vi "Modbus Engine.vi"() -> ()   [LabVIEW 2011]
uses:
  Tushars Events/Software/Modules/EventClient_ObjectReference.ctl
  Strict Type Controls/Settings Operation.ctl
  VIs/MOD bus/nimodbus121/nimodbus121/86/vi.lib/NI Modbus.llb/MB Serial Master Query Write Single Register (poly).vi
  VIs/MOD bus/nimodbus121/nimodbus121/86/vi.lib/NI Modbus.llb/MB Serial Master Query Read Input Registers (poly).vi
panel:
  out "Quit":bool
  out "error out":errorcluster
  in  "error in (no error)":errorcluster
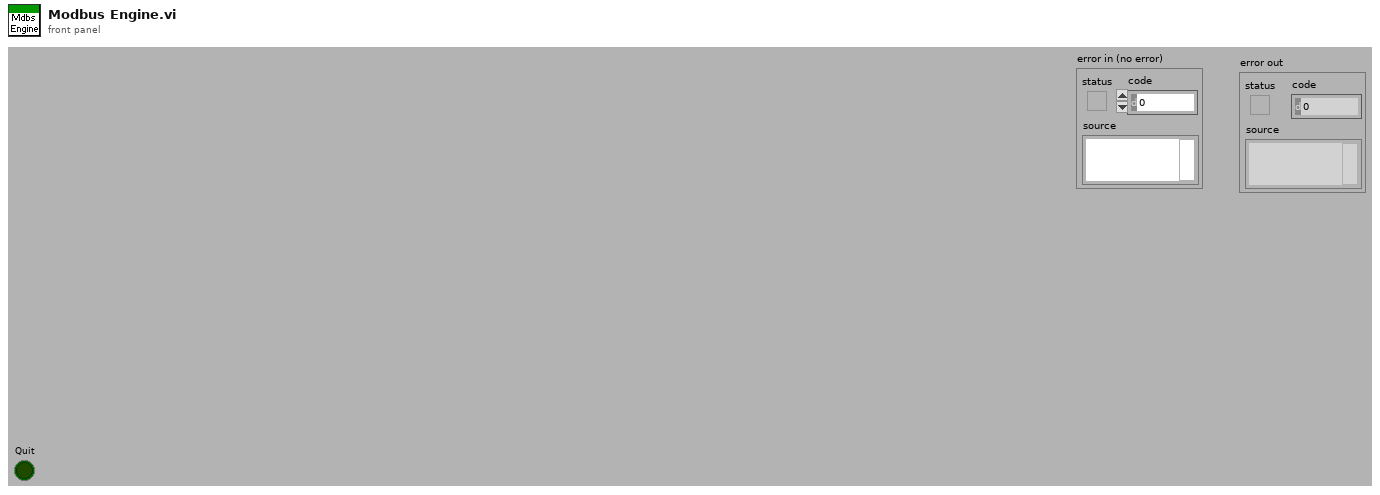
[diagram p1: front panel]
types:
  T1 = typedef "EventClient_ObjectReference.ctl" = refnum<k1>
  T2 = cluster{"Mode":enum16{"RTU", "ASCII"}, "Slave Address":u8}
  T3 = typedef "Settings Operation.ctl" = enum8{"Get Value", "Set Value", "Read File", "Write File", "Write Stored Value"}
  T4 = typedef "Settings.ctl" = cluster{"DMM Settings":cluster{"Port":refnum<visa-resource-name>, "baud rate":u32, "data bits":u16, "stop bits":u16, "parity":enum16{"None", "Odd", "Even", "Mark", "Space"}, "flow control":enum16{"None", "XON/XOFF", "RTS/CTS", "XON/XOFF & RTS/CTS", "DTR/DSR", "XON/XOFF & DTR/DSR"}}, "Modbus Settings":cluster{"Port":refnum<visa-resource-name>, "baud rate":u32, "parity":enum16{"None", "Odd", "Even", "Mark", "Space"}, "flow control":enum16{"None", "XON/XOFF", "RTS/CTS", "XON/XOFF & RTS/CTS", "DTR/DSR", "XON/XOFF & DTR/DSR"}}}
  T5 = enum16{"None", "XON/XOFF", "RTS/CTS", "XON/XOFF & RTS/CTS", "DTR/DSR", "XON/XOFF & DTR/DSR"}
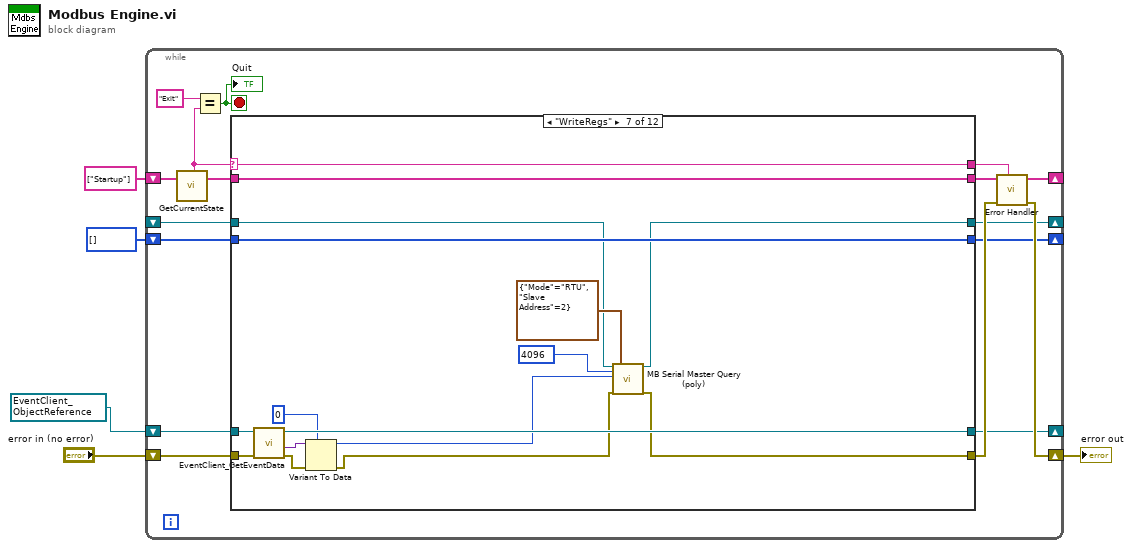
[diagram p0: block diagram]
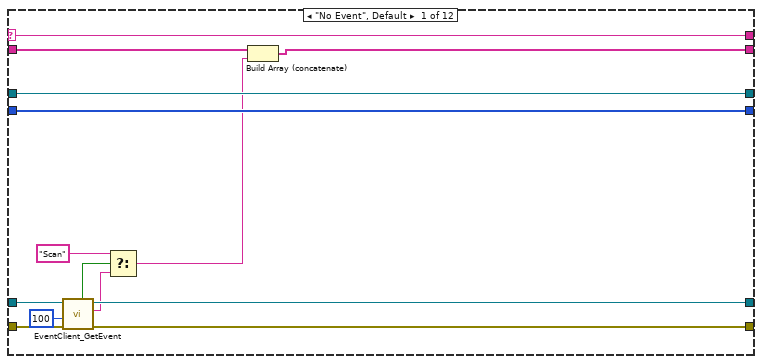
[diagram p2: hidden frame]
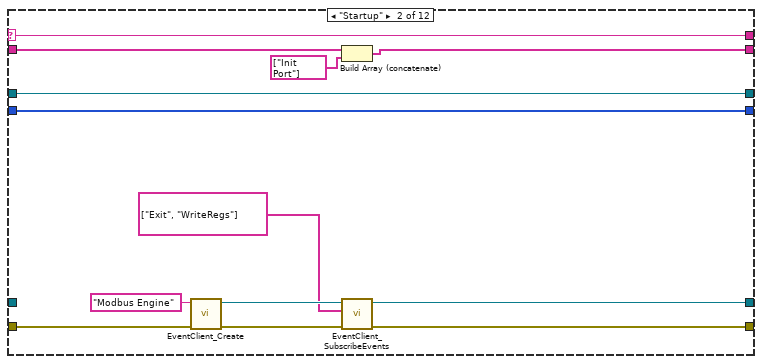
[diagram p3: hidden frame]
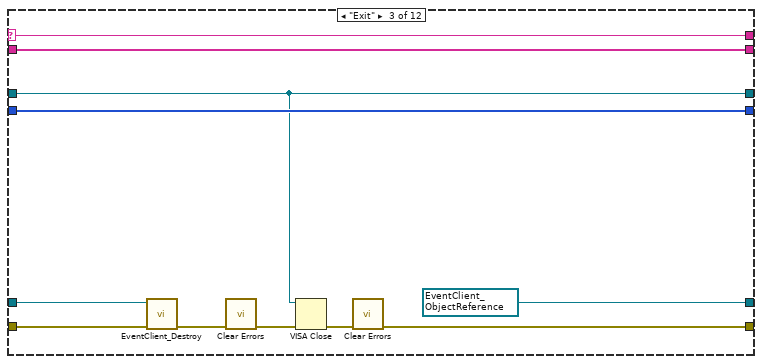
[diagram p4: hidden frame]
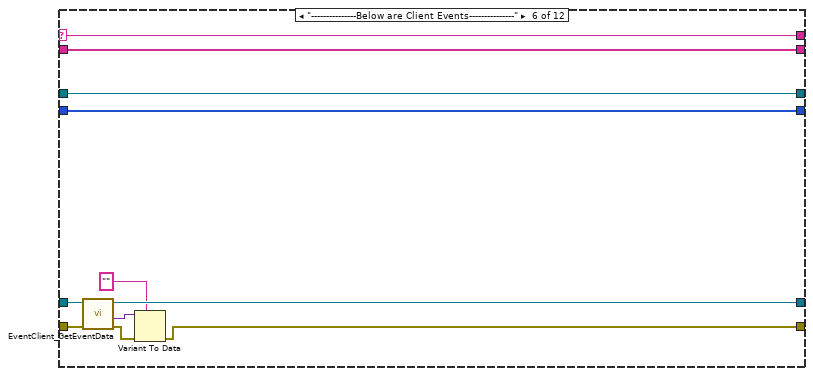
[diagram p7: hidden frame]
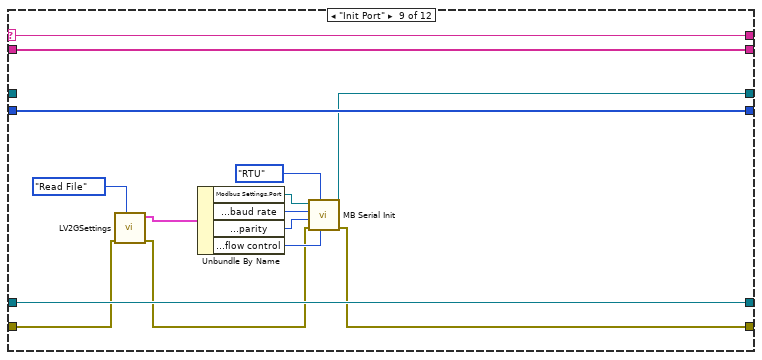
[diagram p9: hidden frame]
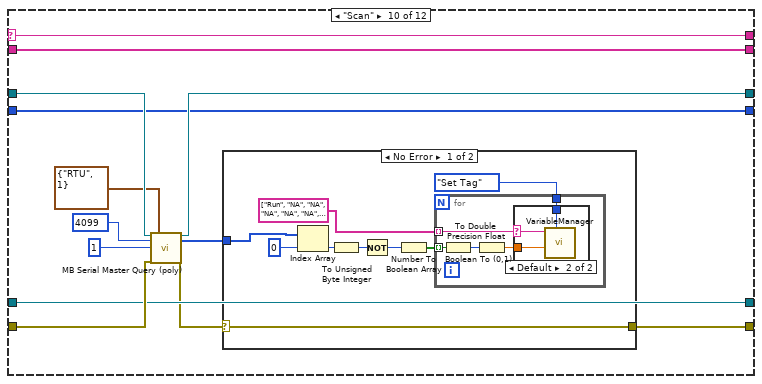
[diagram p10: hidden frame]
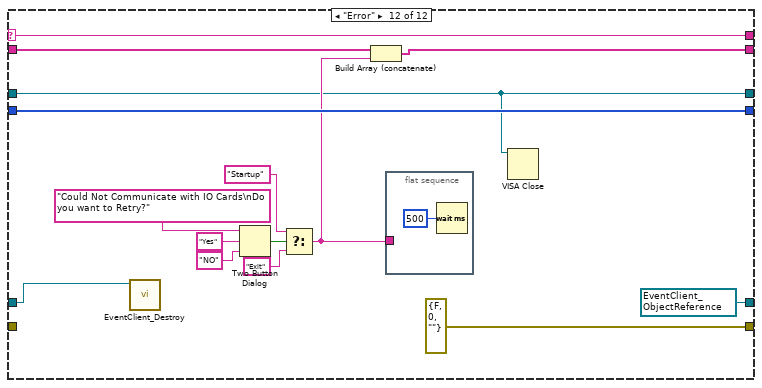
[diagram p14: hidden frame]
diagram:
  w2 = T1 refnum items=["EventClient"] ("reference")
  n1 = while {
    shift-right: [w18] -> _
    shift-left: string[] ["Startup"] ("State Array Out") -> [w22]
    shift-right: [w14] -> w3
    shift-left: "error in (no error)" -> [w15]
    shift-right: [w11] -> _
    shift-left: w2 -> [w10]
    shift-right: [w9] -> _
    shift-left: _ -> [w8]
    shift-right: [w6] -> _
    shift-left: u8[] [] -> [w7]
    stop <- w19 stop-if-true
    n2 = call "GetCurrentState.vi"("State Array In"=w22) -> ("Current State"=w12:string, "State Array Out"=w21:string[])  [unwired: 1 in, 16 out]
    n3 = Equal?(x="Exit", y=w12) -> (x = y?=w19:bool)
    "Quit" <- w19
    n4 = case shown="\"WriteRegs\"" w12 {
      selector: w12 -> [w36 w49 w60 w65 w71 w82 w98 w104 w119 w132 w157 w172]
      tunnel: w21 -> [w29 w48 w59 w66 w72 w83 w99 w105 w120 w133 w156 w163]
      tunnel: [w31 w47 w59 w66 w72 w83 w99 w105 w120 w133 w156 w162] -> w17
      tunnel: [w33 w43 w50 w64 w70 w78 w86 w103 w108 w121 w155 errorcluster {"status"=FALSE, "code"=0, "source"=""} ("error in (no error)")] -> w13
      tunnel: [w36 w49 w60 w65 w71 w82 w98 w104 w119 w132 w157 w172] -> w16
      tunnel: w15 -> [w34 w45 w57 w64 w70 w80 w96 w103 w117 w130 w155 _]
      tunnel: [w32 w41 w56 w63 w69 w76 w93 w102 w118 w129 w154 w159] -> w11
      tunnel: w10 -> [w35 _ w58 w63 w69 w81 w97 w102 w118 w129 w154 w160]
      tunnel: [w28 w38 w54 w62 w68 w75 w84 w101 w110 w128 w153 w158] -> w9
      tunnel: w8 -> [w28 w38 w54 w62 w68 w75 w85 w101 _ w131 w153 w158]
      tunnel: w7 -> [w27 w37 w55 w61 w67 w74 w92 w100 w114 w127 w152 w170]
      tunnel: [w27 w37 w55 w61 w67 w74 w92 w100 w114 w127 w152 w170] -> w6
      frame "No Event", Default {
        n5 = call "EventClient_GetEvent.vi"("error in (no error)"=w34, "timeout in ms (-1)"=100, "reference"=w35) -> ("error out"=w33:errorcluster, "Name"=w24:string, "reference out"=w32:T1, "timed out?"=w26:bool)  [unwired: 5 out]
        n6 = Select(t="Scan" ("x"), s=w26, f=w24) -> (s? t:f=w23:string)
        n7 = Build Array (concatenate)(w29, w23) -> (w31:string[])
      }
      frame "Startup" {
        n8 = call "EventClient_Create.vi"("error in (no error)"=w45, "Instance Name"="Modbus Engine") -> ("error out"=w44:errorcluster, "reference"=w42:T1)  [unwired: 8 out]
        n9 = Build Array (concatenate)(w48, string[] ["Init Port"] ("State Array Out")) -> (w47:string[])
        n10 = call "EventClient_SubscribeEvents.vi"("error in (no error)"=w44, "Events"=string[] ["Exit", "WriteRegs"], "reference"=w42) -> ("error out"=w43:errorcluster, "reference out"=w41:T1)  [unwired: 7 out]
      }
      frame "Exit" {
        w56 = T1 refnum items=["EventClient"] ("reference out")
        n11 = call "EventClient_Destroy.vi"("error in (no error)"=w57, "reference"=w58) -> ("error out"=w53:errorcluster)  [unwired: 9 out]
        n12 = call <vilib>:"Clear Errors.vi"("error in (no error)"=w53) -> ("error out"=w52:errorcluster)  [unwired: 6 out]
        n13 = VISA Close(VISA resource name=w54, error in (no error)=w52) -> (error out=w51:errorcluster)
        n14 = call <vilib>:"Clear Errors.vi"("error in (no error)"=w51) -> ("error out"=w50:errorcluster)  [unwired: 6 out]
      }
      frame "---------------Below are UI Events---------------" {
        # "This State will never Execute\nIt is added just for improving code readability please do not remove this case"
      }
      frame "---------------Below are Menu Events---------------" {
        # "This State will never Execute\nIt is added just for improving code readability please do not remove this case"
      }
      frame "---------------Below are Client Events---------------" {
        n15 = call "EventClient_GetEventData.vi"("error in (no error)"=w80, "reference"=w81) -> ("error out"=w79:errorcluster, "Data"=w77:variant, "reference out"=w76:T1)  [unwired: 7 out]
        n16 = Variant To Data(error in=w79, type="", Variant=w77) -> (error out=w78:errorcluster)  [unwired: 1 out]
      }
      frame "WriteRegs" {
        n17 = call "EventClient_GetEventData.vi"("error in (no error)"=w96, "reference"=w97) -> ("error out"=w95:errorcluster, "Data"=w94:variant, "reference out"=w93:T1)  [unwired: 7 out]
        n18 = Variant To Data(error in=w95, type=u16 0 ("unsigned 16bit integer"), Variant=w94) -> (data=w88:u16, error out=w87:errorcluster)
        n19 = call-poly "MB Serial Master Query (poly).vi"("VISA resource name"=w85, "Address"=u16 4096 ("Starting Address"), "Holding Register"=w88, "error in"=w87, "Serial Parameters"=T2 {"Mode"=enum."RTU", "Slave Address"=2}) -> ("VISA resource name out"=w84:refnum<visa-resource-name>, "error out"=w86:errorcluster)  [unwired: 2 in, 11 out]
      }
      frame "---------------Below are Subroutine states---------------" {
      }
      frame "Init Port" {
        n20 = call "LV2GSettings.vi"("Operation"=Settings_Operation."Read File", "error in (no error)"=w117) -> ("error out"=w109:errorcluster, "Settings out"=w115:T4)  [unwired: 1 in, 7 out]
        n21 = Unbundle By Name(w115) -> ("Modbus Settings.Port"=w106:refnum<visa-resource-name>, "Modbus Settings.baud rate"=w113:u32, "Modbus Settings.parity"=w112:enum16{"None", "Odd", "Even", "Mark", "Space"}, "Modbus Settings.flow control"=w111:T5)
        n22 = call "MB Serial Init.vi"("Flow Control"=w111, "Mode"=enum16{"RTU", "ASCII"}."RTU", "error in (no error)"=w109, "Parity"=w112, "Baud Rate"=w113, "VISA resource name"=w106) -> ("error out"=w108:errorcluster, "VISA resource name out"=w110:refnum<visa-resource-name>)  [unwired: 1 in, 3 out]
      }
      frame "Scan" {
        n23 = call-poly "MB Serial Master Query (poly).vi"("VISA resource name"=w131, "Starting Address"=u16 4099, "Quantity"=u16 1, "error in"=w130, "Serial Parameters"=T2 {"Mode"=enum."RTU", "Slave Address"=1}) -> ("VISA resource name out"=w128:refnum<visa-resource-name>, "Input Registers"=w124:u16[], "error out"=w122:errorcluster)  [unwired: 2 in, 10 out]
        n24 = case shown="No Error" w122 {
          selector: w122 -> [w134 w151]
          tunnel: w124 -> [w142 _]
          tunnel: [w134 w151] -> w121
          frame No Error {
            n25 = Index Array(array=w142, index=0) -> (element=w140:u16)
            n26 = To Unsigned Byte Integer(number=w140) -> (unsigned 8bit integer=w139:u8)
            n27 = Not(x=w139) -> (.not. x?=w135:u8)
            n28 = Number To Boolean Array(number=w135) -> (Boolean array=w138:bool[])
            n29 = for {
              tunnel: w138 -> [w147] mode=indexing
              tunnel: string[] ["Run", "NA", "NA", "NA", "NA", "NA", "NA", "NA"] -> [w144] mode=indexing
              tunnel: enum16{"Get Tag", "Set Tag"}."Set Tag" ("Operation") -> [w143]
              n30 = Boolean To (0,1)(Boolean=w147) -> (0, 1=w146:i16)
              n31 = To Double Precision Float(number=w146) -> (double precision float=w145:dbl)
              n32 = case shown="Default" w144 {
                selector: w144 -> [_ w149]
                tunnel: w145 -> [_ w150]
                tunnel: w143 -> [_ w148]
                frame "", "NA" {
                }
                frame Default {
                  n33 = call "VariableManager.vi"("Operation"=w148, "Value"=w150, "Tag"=w149) -> ()  [unwired: 9 out]
                }
              }
            }
          }
          frame Error {
          }
        }
      }
      frame "---------------Below are Error Handling VIs---------------" {
      }
      frame "Error" {
        w159 = T1 refnum items=["EventClient"] ("reference")
        n34 = call "EventClient_Destroy.vi"("reference"=w160) -> ()  [unwired: 1 in, 10 out]
        n35 = Two Button Dialog(message="Could Not Communicate with IO Cards\nDo you want to Retry?", 1:"NO" ("F button name (\"Cancel\")"), 2:"Yes" ("T button name (\"OK\")")) -> (T button?=w167:bool)
        n36 = Select(t="Startup" ("String"), s=w167, f="Exit" ("String")) -> (s? t:f=w161:string)
        n37 = Build Array (concatenate)(w163, w161) -> (w162:string[])
        n38 = flat-sequence {
          tunnel: w161 -> [_]
          frame #0 {
            n39 = Wait (ms)(milliseconds to wait=u32 500) -> ()  [unwired: 1 out]
          }
        }
        n40 = VISA Close(VISA resource name=w158) -> ()  [unwired: 1 in, 1 out]
      }
    }
    n41 = call "Error Handler.vi"("Current State"=w16, "error in (no error)"=w13, "Msg Queue In"=w17) -> ("error out"=w14:errorcluster, "Msg Queue Out"=w18:string[])  [unwired: 1 in, 6 out]
  }
  "error out" <- w3
